vi "simulated_g=1.vi"() -> ()   [LabVIEW 2016]
panel:
  out "trion 2":cluster{dbl[], dbl[]}[](graph)=[{[3.5, 3.75, 4.0, 4.25, 4.5, 4.75, 5.0, 5.25, 5.5, 5.75, 6.0, 6.25, 6.5, 6.75, 7.0, 7.25, 7.5], [0.09884225881608028, 0.08311363983983036, 0.06905018843369463, 0.05482590567191773, 0.040548882893517685, 0.026455307876812634, 0.010354155742091748, 0.002573870467875914, 0.016815129240448104, 0.03115684059448202, 0.04541261541184766, 0.059701047845767484, 0.0740328904177516, 0.08837518579897312, 0.10262200649225614, 0.11695375221889187, 0.1307608718110925]}]
  out "pair 2":cluster{dbl[], dbl[]}[](graph)=[{[2.75, 3.0, 3.25, 3.5, 3.75, 4.0, 4.25, 4.5, 4.75, 5.0, 5.25, 5.5, 5.75, 6.0, 6.25, 6.5, 6.75, 7.0, 7.25, 7.5, 7.75], [0.10161861073779858, 0.0913983764190916, 0.08122555457233184, 0.07107879079479013, 0.060888414576019324, 0.05069977391553355, 0.04051875023908746, 0.03030289534240021, 0.020208917910533353, 0.007280699439795031, 3.1945405346242573e-07, 0.010609776939633796, 0.020753686237935547, 0.030905054478379334, 0.0410618225265827, 0.051254331232383335, 0.06142685083884415, 0.07163587276239983, 0.08179930205992073, 0.09198757001428791, 0.10216932294440752]}]
  out "widths":cluster{dbl[], dbl[]}[](graph)
  out "amplitudes":cluster{dbl[], dbl[]}[](graph)
  in  "trion":cluster{dbl[], dbl[]}(graph)
  in  "pair":cluster{dbl[], dbl[]}(graph)
  in  "fits 2":cluster{dbl[], dbl[]}[](graph)
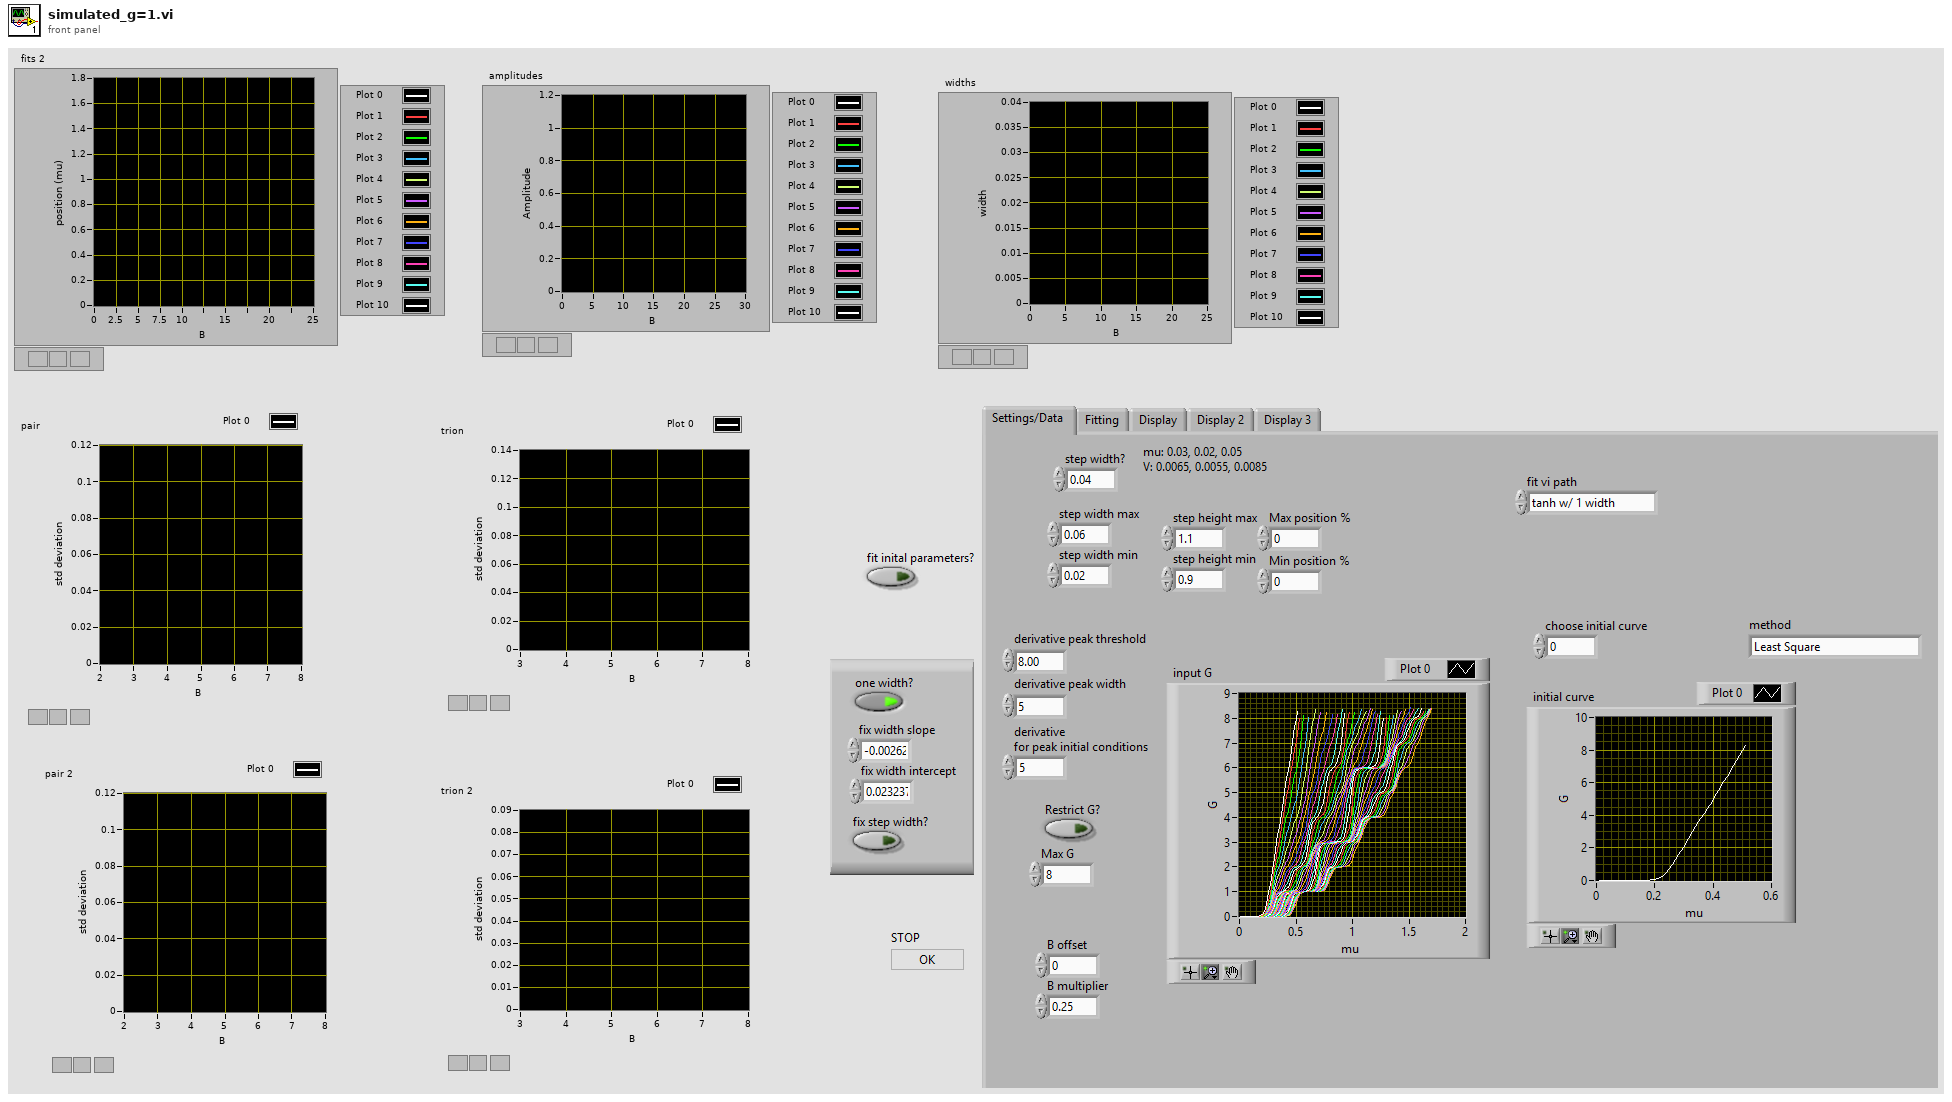
[diagram p1: front panel]
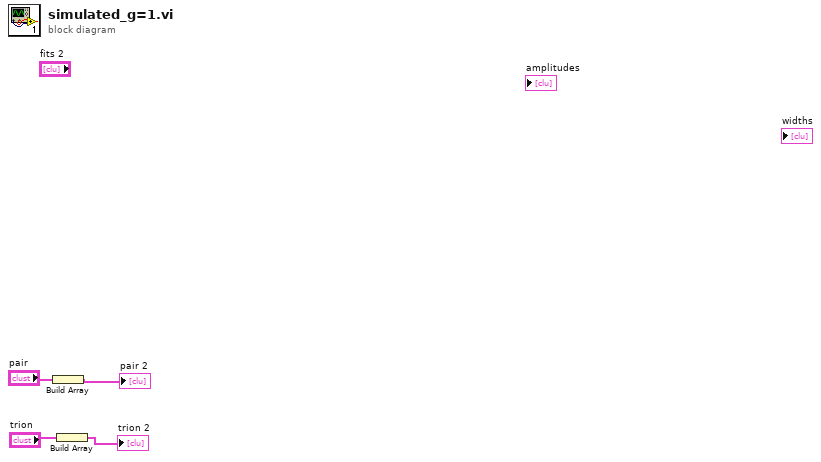
[diagram p0: block diagram]
diagram:
  n1 = Build Array("pair") -> (→"pair 2":cluster{dbl[], dbl[]}[])
  n2 = Build Array("trion") -> (→"trion 2":cluster{dbl[], dbl[]}[])
